vi "GV retrigger.vi"() -> ()   [LabVIEW 2016]
panel:
  in  "Re-trigger":bool
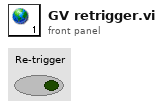
[diagram p1: front panel]
diagram:
